vi "IncludeProjectLibrary_IgnoreItemsInPrivateScope_WhitelistNotContainsFile.vi"(9 "file":path) -> (0 "error out":errorcluster)   [LabVIEW 2017, in "Whitelist.Tests.lvlib"]
uses:
  Whitelist.Tests.lvlib
  Whitelist/Whitelist.lvclass
  Assertion/Assertion.lvlib
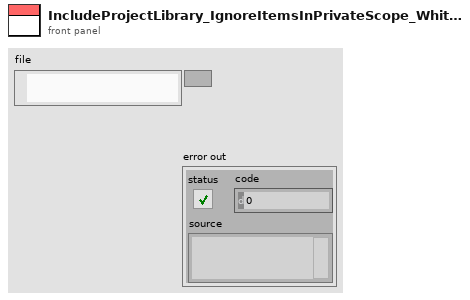
[diagram p1: front panel]
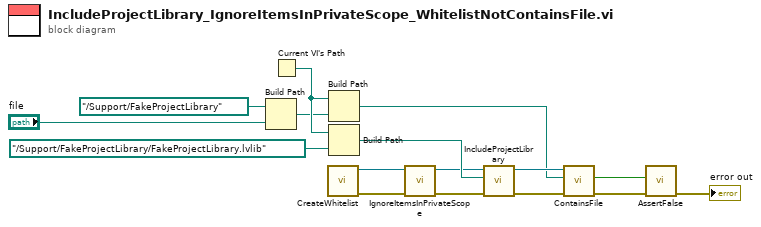
[diagram p0: block diagram]
diagram:
  n1 = Build Path(base path=path "../Support/FakeProjectLibrary", name or relative path="file") -> (appended path=w5:path)
  n2 = Current VI's Path() -> (path=w9:path)
  n3 = call "CreateWhitelist.vi"() -> ("error out"=w16:errorcluster, "Whitelist out"=w2:refnum<class "Whitelist.lvclass">)  [unwired: 10 in]
  n4 = Build Path(base path=w9, name or relative path=w5) -> (appended path=w8:path)
  n5 = Build Path(base path=w9, name or relative path=path "../Support/FakeProjectLibrary/FakeProjectLibrary.lvlib" ("relative_library_path")) -> (appended path=w10:path)
  n6 = call "IgnoreItemsInPrivateScope.vi"("error in (no error)"=w16, "Whitelist in"=w2) -> ("error out"=w3:errorcluster, "Whitelist out"=w1:refnum<class "Whitelist.lvclass">)  [unwired: 8 in]
  n7 = call "IncludeProjectLibrary.vi"("error in (no error)"=w3, "Path"=w10, "Whitelist in"=w1) -> ("error out"=w14:errorcluster, "Whitelist out"=w15:refnum<class "Whitelist.lvclass">)  [unwired: 7 in]
  n8 = call "ContainsFile.vi"("error in (no error)"=w14, "Path"=w8, "Whitelist in"=w15) -> ("error out"=w13:errorcluster, "Is Whitelisted?"=w12:bool)  [unwired: 6 in, 1 out]
  n9 = call "AssertFalse.vi"("error in (no error)"=w13, "Condition"=w12) -> ("error out"=→"error out":errorcluster)  [unwired: 9 in]
